vi "Get or Register Entity.vi"(10 "Entity":refnum<class "Entity.lvclass">, 11 "Entity Manager in":refnum<class "Entity Manager.lvclass">) -> (1 "Entity Info":T1, 3 "Entity Manager out":refnum<class "Entity Manager.lvclass">)   [LabVIEW 2020, in "Conditu2.lvlib" / "Entity Manager.lvclass"]
uses:
  Entity Manager.lvclass
  Entity/Entity.lvclass
  Known Entity.ctl
  Columns/Type/Type.lvclass
  Entity Manager.lvclass/Entity Manager.ctl
  Columns/Type/Type.lvclass/Type.ctl
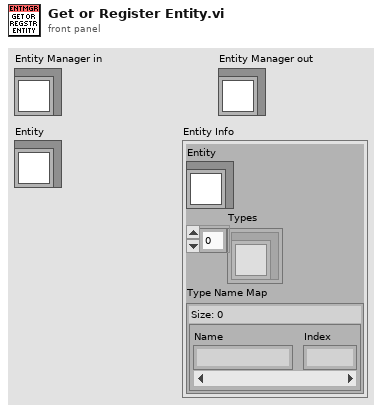
[diagram p1: front panel]
types:
  T1 = typedef "Conditu2.lvlib/Entity Manager.lvclass/Known Entity.ctl" = cluster{"Entity":refnum<class "Entity.lvclass">, "Types":refnum<class "Type.lvclass">[], "Type Name Map":map{string, i32}}
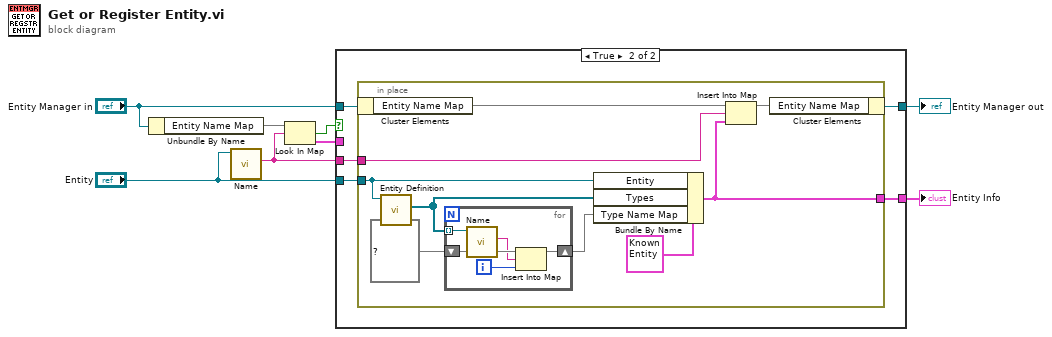
[diagram p0: block diagram]
diagram:
  n1 = Unbundle By Name("Entity Manager in") -> ("Entity Name Map"=w7:map{string, T1})
  n2 = call-dynamic "Name.vi"("Entity in"="Entity") -> ("Name"=w5:string)  [unwired: 10 in]
  n3 = Look In Map(map=w7, key=w5) -> (key not found?=w4:bool, value=w3:T1)  [unwired: 1 in]
  n4 = case shown="True" w4 {
    tunnel: "Entity Manager in" -> [w10 w15]
    tunnel: "Entity" -> [_ w14]
    tunnel: w5 -> [_ w13]
    tunnel: w3 -> [w9 _]
    tunnel: [w10 w12] -> w2
    tunnel: [w9 w11] -> w1
    frame False {
    }
    frame True {
      n5 = in-place {
        in-place-border: w14 -> [w19]
        in-place-border: w13 -> [w22]
        in-place-border: [w16] -> w11
        n6 = in-place-cluster #1(w15) -> ("Entity Name Map"=w24:map{string, T1})
        n7 = call "Entity Definition.vi"("Entity in"=w19) -> ("Definition"=w17:refnum<class "Type.lvclass">[])  [unwired: 10 in]
        n8 = for {
          tunnel: w17 -> [w29] mode=indexing
          shift-right: [w25] -> w18
          shift-left: map{string, i32} {} ("Type Name Map") -> [w28]
          i -> [w26]
          n9 = call "Name.vi"("Type in"=w29) -> ("Table Name"=w27:string)  [unwired: 10 in]
          n10 = Insert Into Map(map in=w28, key=w27, value=w26) -> (map out=w25:map{string, i32})  [unwired: 2 out]
        }
        n11 = Bundle By Name(cluster=T1 {"Entity"=refnum, "Types"=[], "Type Name Map"={}} ("Known Entity"), "Entity"=w19, "Types"=w17, "Type Name Map"=w18) -> (w16:T1)
        n12 = Insert Into Map(map in=w24, key=w22, value=w16) -> (map out=w23:map{string, T1})  [unwired: 2 out]
        n13 = in-place-cluster #1("Entity Name Map"=w23) -> (w12:refnum<class "Entity Manager.lvclass">)
      }
    }
  }
  "Entity Manager out" <- w2
  "Entity Info" <- w1
